vi "Launch Measurement and Wait for Result.vi"(8 "error in (no error)":errorcluster, 11 "Launch Measurement and Wait for Result in":refnum<class "Launch Measurement and Wait for Result.lvclass">) -> (0 "error out":errorcluster, 3 "Launch Measurement and Wait for Result out":refnum<class "Launch Measurement and Wait for Result.lvclass">)   [LabVIEW 2016, in "Controller API.lvlib" / "Launch Measurement and Wait for Result.lvclass"]
uses:
  <userlib>/Measurement Utility API/Messages/Launch Measurement Msg/Launch Measurement and Wait for Result.lvclass
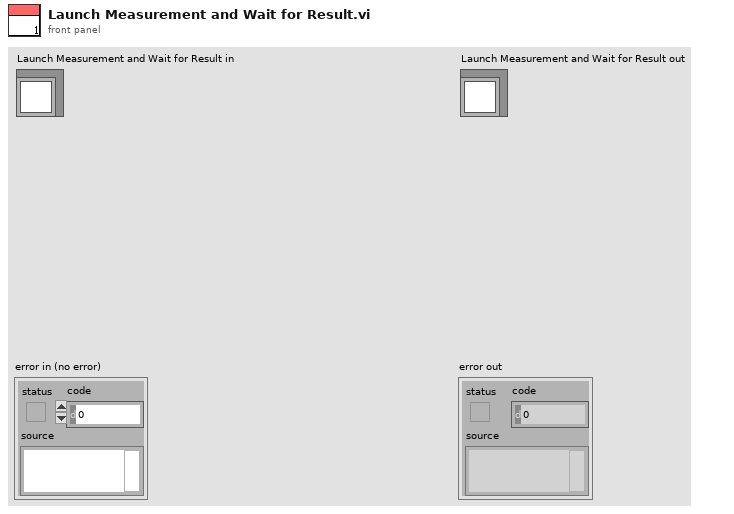
[diagram p1: front panel]
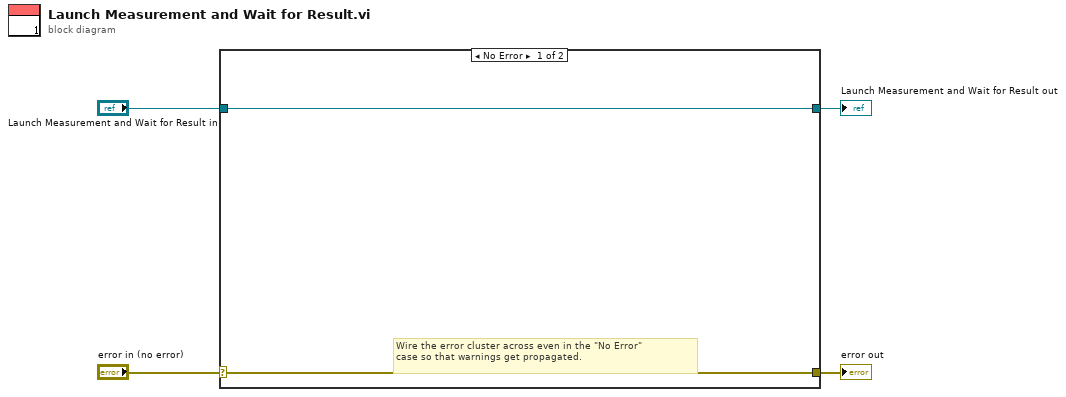
[diagram p0: block diagram]
diagram:
  n1 = case shown="No Error" "error in (no error)" {
    selector: "error in (no error)" -> [w5 w8]
    tunnel: [w5 w8] -> w3
    tunnel: [w6 w7] -> w1
    tunnel: "Launch Measurement and Wait for Result in" -> [w6 w7]
    frame No Error {
      # "Wire the error cluster across even in the \"No Error\"\ncase so that warnings get propagated."
    }
    frame Error {
    }
  }
  "error out" <- w3
  "Launch Measurement and Wait for Result out" <- w1
